vi "ton.vi"(8 "reference":refnum<vi>, 10 "Time":i32, 11 "START":bool) -> (2 "ET":i32, 3 "Q":bool)   [LabVIEW 2020]
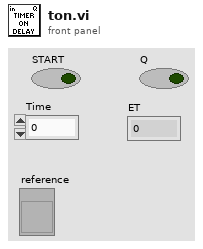
[diagram p1: front panel]
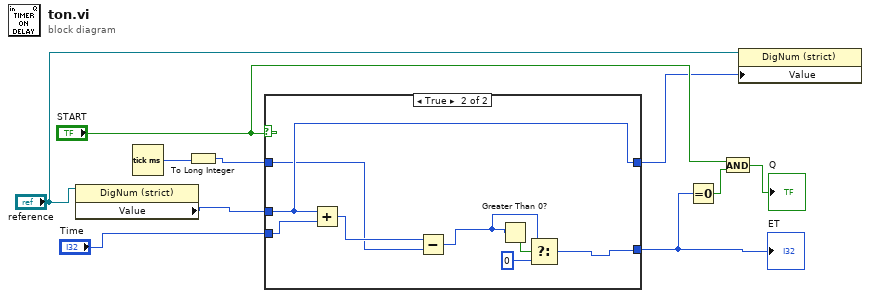
[diagram p0: block diagram]
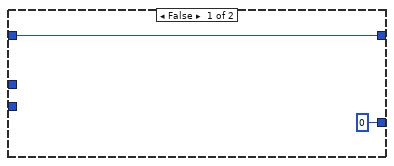
[diagram p2: hidden frame]
diagram:
  n1 = property class="DigNum (strict)"(reference="reference") -> ("Value"=w3:i32)  [unwired: 1 in, 2 out]
  n2 = Tick Count (ms)() -> (millisecond timer value=w6:u32)
  n3 = To Long Integer(number=w6) -> (32bit integer=w5:i32)
  n4 = case shown="True" "START" {
    tunnel: w5 -> [w12 w17]
    tunnel: [w12 w20] -> w2
    tunnel: w3 -> [_ w20]
    tunnel: "Time" -> [_ w19]
    tunnel: [0 ("f") w14] -> w4
    frame False {
    }
    frame True {
      n5 = Add(x=w20, y=w19) -> (x+y=w18:i32)
      n6 = Subtract(x=w18, y=w17) -> (x-y=w15:i32)
      n7 = Greater Than 0?(x=w15) -> (x > 0?=w16:bool)
      n8 = Select(t=w15, s=w16, f=0) -> (s? t:f=w14:i32)
    }
  }
  "ET" <- w4
  n9 = Equal To 0?(x=w4) -> (x = 0?=w8:bool)
  n10 = And(x="START", y=w8) -> (x .and. y?=→"Q":bool)
  n11 = property class="DigNum (strict)"(reference="reference", "Value"=w2) -> ()  [unwired: 1 in, 2 out]
